vi "Generate write queue item.vi"(8 "error in (no error)":errorcluster, 9 "Registration ID":u64, 10 "Request ID":u64, 11 "Unregister JSON in":refnum<class "Unregister JSON.lvclass">) -> (0 "error out":errorcluster, 2 "Write queue item":T1, 3 "Unregister JSON out":refnum<class "Unregister JSON.lvclass">)   [LabVIEW 2020, in "wamplv.lvlib" / "Unregister JSON.lvclass"]
uses:
  Unregister JSON.lvclass
  Unregister JSON.lvclass/Unregister JSON.ctl
  wamplv.lvlib
  b16c139c-bd7d-4c5b-afdf-b796f9a4fff9.vi
  TypeDefs/WAMP Message Codes.ctl
  TypeDefs/Transport type.ctl
  WAMP Client/Private/TypeDef/Write queue item.ctl
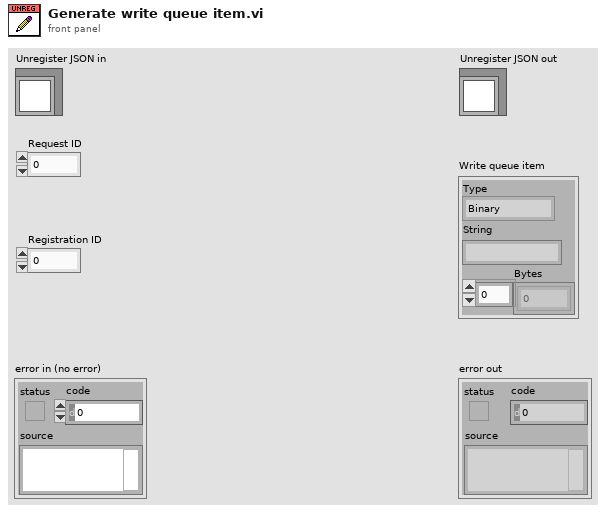
[diagram p1: front panel]
types:
  T1 = typedef "wamplv.lvlib/Write queue item.ctl" = cluster{"Type":T2, "String":string, "Bytes":u8[]}
  T2 = typedef "wamplv.lvlib/Transport type.ctl" = enum16{"Binary", "Text"}
  T3 = typedef "wamplv.lvlib/WAMP Message Codes.ctl" = enum8{"HELLO", "WELCOME", "ABORT", "GOODBYE", "ERROR", "PUBLISH", "PUBLISHED", "SUBSCRIBE", "SUBSCRIBED", "UNSUBSCRIBE", "UNSUBSCRIBED", "EVENT", "CALL", "RESULT", "REGISTER", "REGISTERED", "UNREGISTER", "UNREGISTERED", "INVOCATION", "YIELD"}
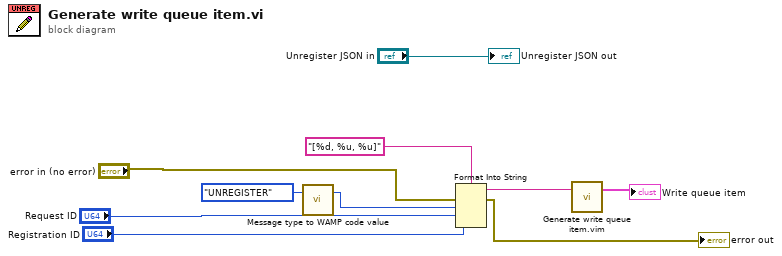
[diagram p0: block diagram]
diagram:
  n1 = call "Message type to WAMP code value.vi"("Message Type"=WAMP_Message_Codes."UNREGISTER") -> ("WAMP Numeric value"=w2:u8)  [unwired: 2 in]
  n2 = Format Into String(format string="[%d, %u, %u]" ("element"), error in="error in (no error)", w2, "Request ID", "Registration ID") -> (resulting string=w4:string, error out=→"error out":errorcluster)  [unwired: 1 in]
  n3 = call "Generate write queue item.vim"("Input"=w4) -> ("Ouput"=→"Write queue item":T1)  [unwired: 2 in]
  "Unregister JSON out" <- "Unregister JSON in"
